vi "FlickerEventCallback.vi"(4 "?":refnum<vi>, 5 "Event Data":cluster{"sender":refnum<k24>, "e":refnum<k24>}, 6 "Control Ref":refnum<k24>, 7 "Event Common Data":T1) -> ()   [LabVIEW 2014]
uses:
  C:/Users/ThomasNelson/Projects/examples/libraries/bin/visual .net/KClmtrWrapper.dll
  libraries/bin/visual .net/KClmtrWrapper.dll
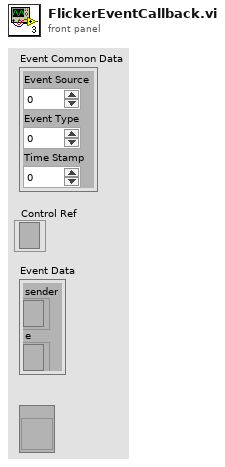
[diagram p1: front panel]
types:
  T1 = cluster{"Event Source":i32, "Event Type":u32, "Time Stamp":u32}
  T2 = cluster{"dB Graph":cluster{"X":dbl, "Y":dbl}[], "big Y":dbl}
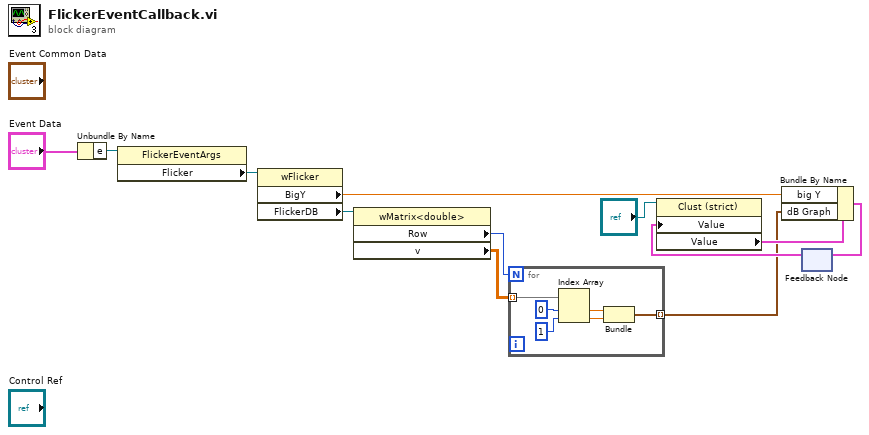
[diagram p0: block diagram]
diagram:
  n1 = Unbundle By Name("Event Data") -> ("e"=w7:refnum<k24>)
  n2 = property class="FlickerEventArgs"(reference=w7) -> ("Flicker"=w6:refnum<k24>)  [unwired: 1 in, 2 out]
  n3 = property class="wFlicker"(reference=w6) -> ("BigY"=w1:dbl, "FlickerDB"=w5:refnum<k24>)  [unwired: 1 in, 2 out]
  n4 = property class="wMatrix<double>"(reference=w5) -> ("Row"=w4:i32, "v"=w3:dbl[][])  [unwired: 1 in, 2 out]
  n5 = for {
    N: w4 -> [_]
    tunnel: w3 -> [w18] mode=indexing
    tunnel: [w13] -> w2 mode=indexing
    n6 = Index Array(array=w18, index #1=0 ("index"), index #2=1 ("index")) -> (element #1=w15:dbl, element #2=w14:dbl)
    n7 = Bundle(w15, w14) -> (w13:cluster{dbl, dbl})  [unwired: 1 in]
  }
  n8 = feedback #1() -> (w10:T2)  [unwired: 1 in]
  n9 = property class="Clust (strict)"(reference="?", "Value"=w10) -> ("Value"=w8:T2)  [unwired: 1 in, 2 out]
  n10 = Bundle By Name(cluster=w8, "big Y"=w1, "dB Graph"=w2) -> (w11:T2)
  n11 = feedback-in #1(w11) -> ()
